vi "Dereference-PointerOfPointer.vi"(8 "No Error":errorcluster, 11 "Ptr of Ptr [void **]":i64 format="%.0x") -> (0 "error out":errorcluster, 3 "Ptr [void *]":i64)   [LabVIEW 2026, in "SDL3.lvlib" / "LV-Utilities.lvlib"]
doc: "<B>Summary</B>\nDereference pointer of pointer into pointer."
uses:
  LV-Utilities.lvlib
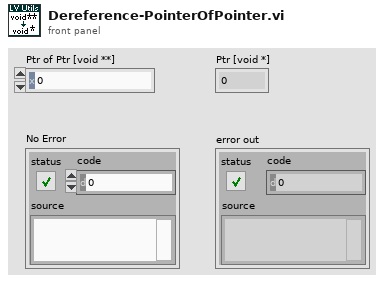
[diagram p1: front panel]
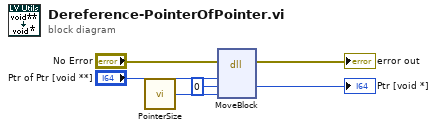
[diagram p0: block diagram]
diagram:
  n1 = call "PointerSize.vi"() -> ("Pointer Size [Byte]"=w2:i32)
  n2 = dll-call lib="LabVIEW" fn="MoveBlock"(error in="No Error", "Address"="Ptr of Ptr [void **]", "Destination"=i64 0, "Size"=w2) -> (error out=→"error out":errorcluster, "Destination"=→"Ptr [void *]":i64)  [unwired: 5 in, 1 out]
